vi "Choose Implementation Dialog.vi"(8 "error in (no error)":errorcluster, 9 "DNL_Activate BD":bool, 10 "Method Name":string, 11 "DNL_Wired Class Refnum":refnum<vi>) -> (0 "error out":errorcluster, 2 "Class Hierarchy":string[](array[string]), 3 "DNL_Wired Class Refnum out":refnum<vi>)   [LabVIEW 2020, in "Choose Implementation Dialog.lvlib"]
uses:
  Choose Implementation Dialog.lvlib
  da94b13a-eb72-4d8b-8881-ae04a75001f9.vi
panel:
  in  "format string":string="Error %d while initializing Choose Implementation dialog."
  in  "Class Hierarchy":string[](tree) caption="Select VI"
  in  "Help":bool
  in  "Cancel":bool
  in  "Open":bool
  # "* You can Ctrl-click multiple items in the list to open multiple method VIs."
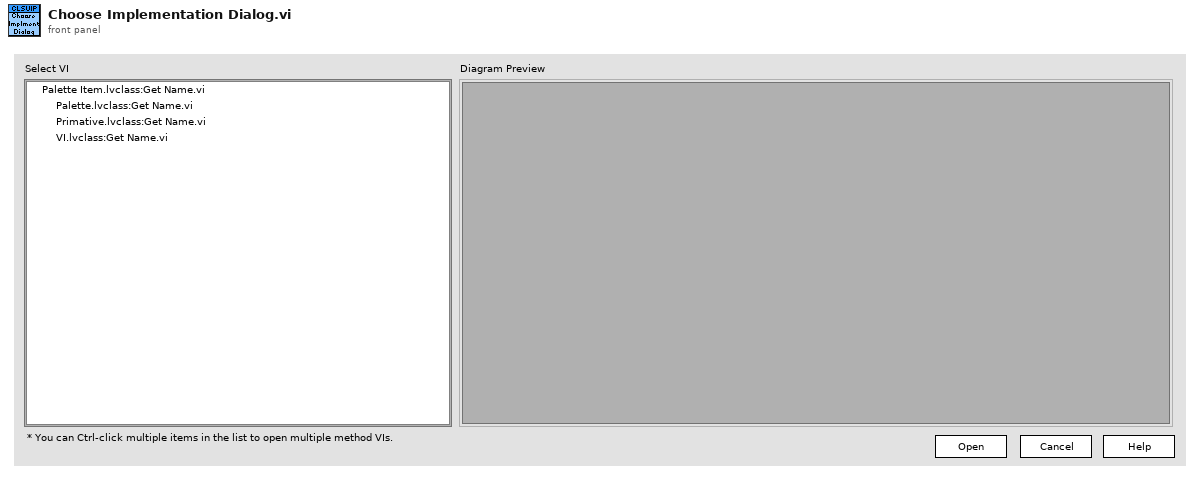
[diagram p1: front panel]
types:
  T1 = typedef "LVPointTypeDef.ctl" = cluster{"Horizontal":i16, "Vertical":i16}
  T2 = typedef "LVRectTypeDef.ctl" = cluster{"Left":i16, "Top":i16, "Right":i16, "Bottom":i16}
  T3 = typedef "LVPoint32TypeDef.ctl" = cluster{"Horizontal":i32, "Vertical":i32}
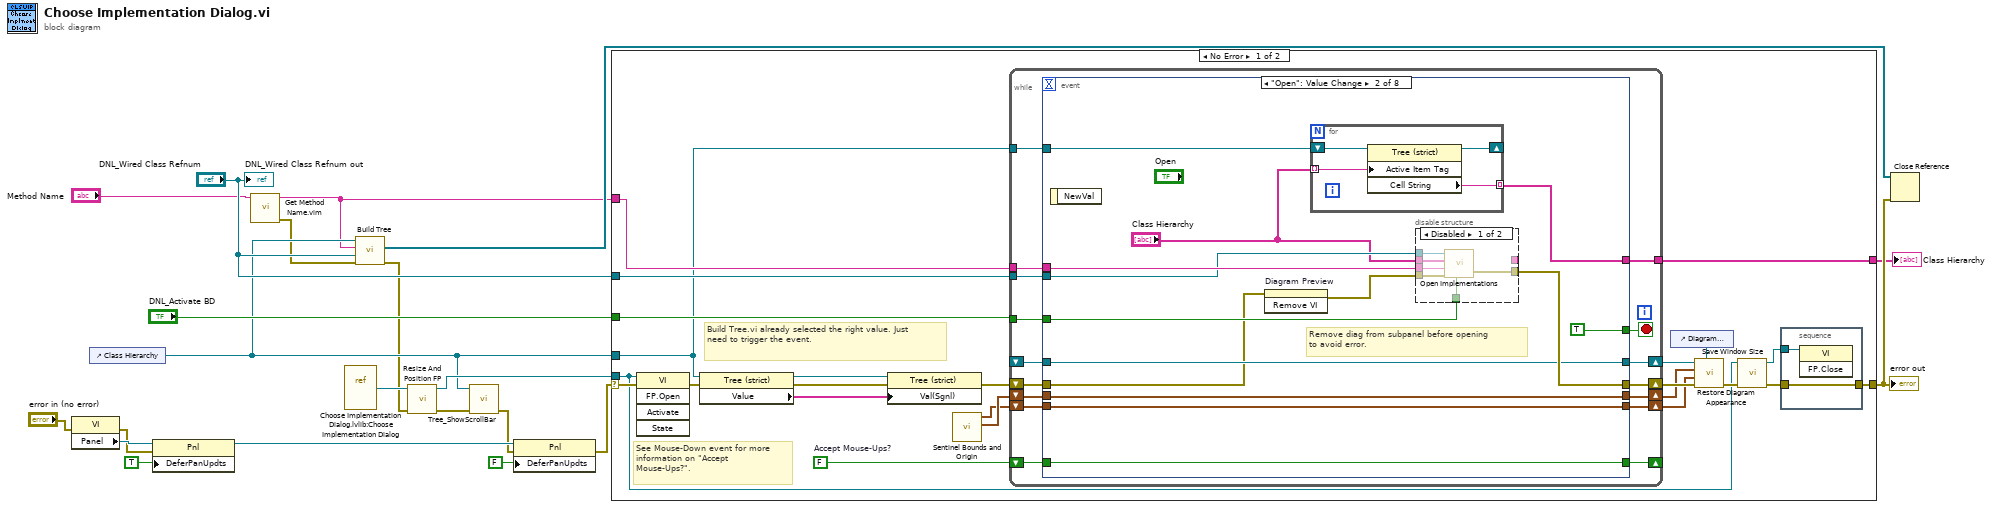
[diagram p0: block diagram]
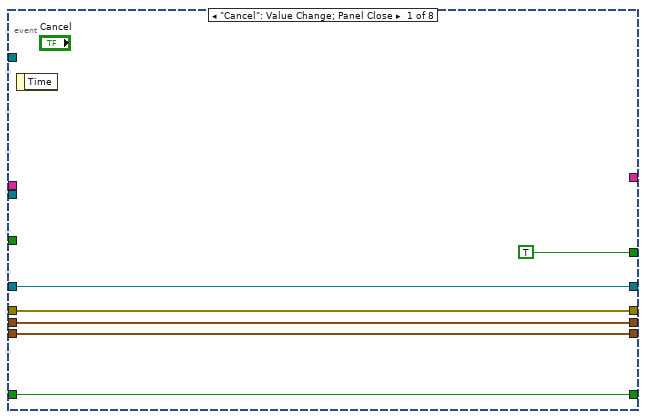
[diagram p2: hidden frame]
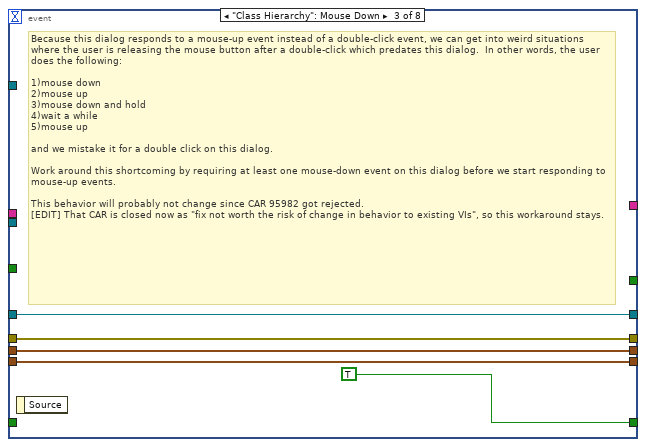
[diagram p4: hidden frame]
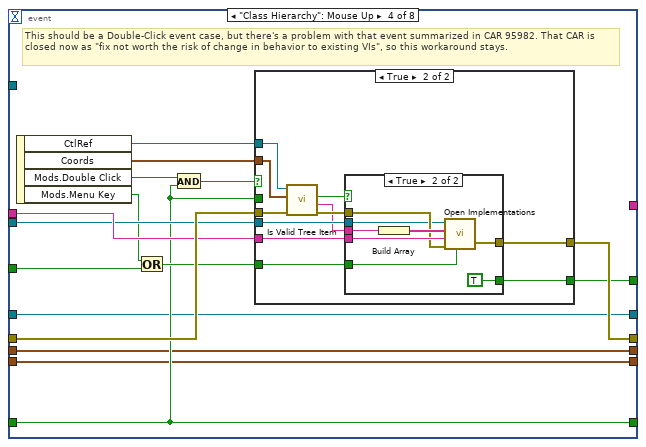
[diagram p5: hidden frame]
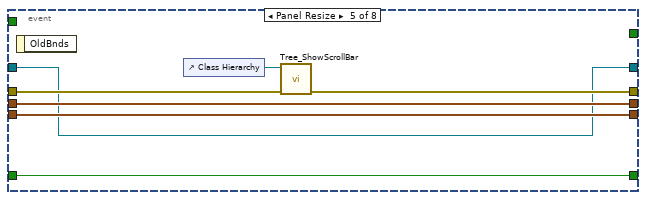
[diagram p8: hidden frame]
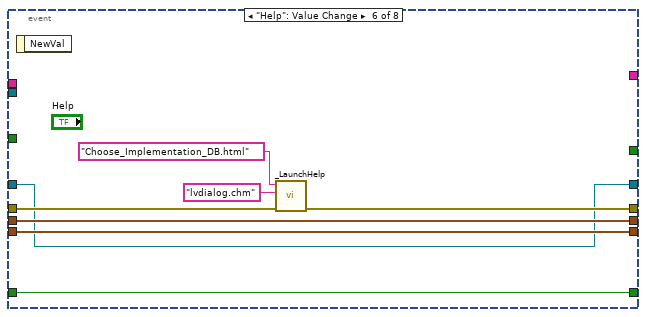
[diagram p9: hidden frame]
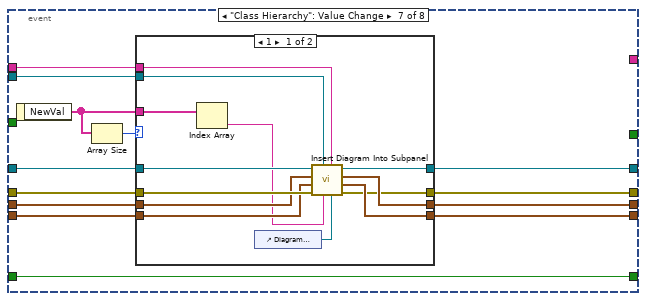
[diagram p10: hidden frame]
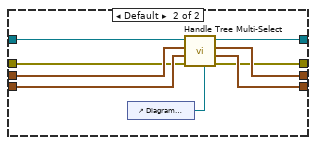
[diagram p11: hidden frame]
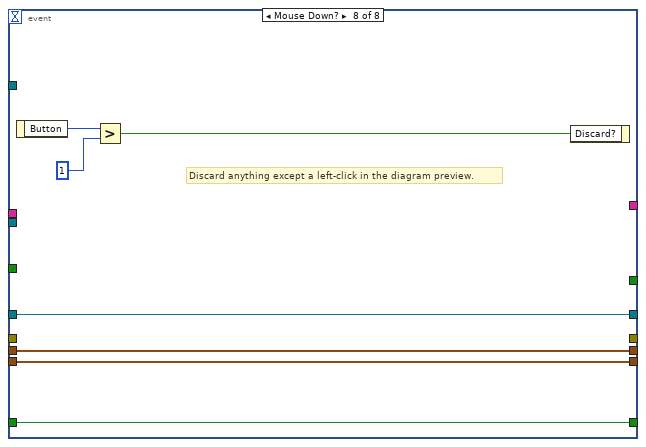
[diagram p12: hidden frame]
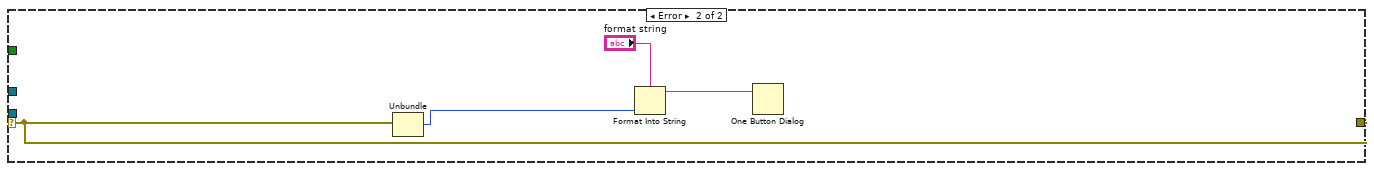
[diagram p13: hidden frame]
diagram:
  n1 = property class="VI"(error in="error in (no error)") -> (error out=w13:errorcluster, "Panel"=w16:refnum<vi>)  [unwired: 1 in, 1 out]
  n2 = control-ref of="Class Hierarchy"() -> (w7:refnum<vi>)
  n3 = property class="Pnl"(reference=w16, error in=w13, "DeferPanUpdts"=TRUE ("Defer Panel Updates")) -> (reference out=w11:refnum<vi>)  [unwired: 1 out]
  n4 = call "Get Method Name.vim"("VI Reference/Name"="Method Name") -> ("error out"=w3:errorcluster, "Method Name"=w2:string)  [unwired: 9 in]
  n5 = vi-ref "Choose Implementation Dialog.lvlib:Choose Implementation Dialog.vi"() -> (w21:refnum<vi>)
  n6 = call "Build Tree.vi"("error in (no error)"=w3, "Wired-in Class Refnum"="DNL_Wired Class Refnum", "Method Name"=w2, "Tree Refnum"=w7) -> ("error out"=w6:errorcluster, "All Classes"=w18:refnum<vi>[])  [unwired: 6 out]
  n7 = call "Resize And Position FP.vi"("error in (no error)"=w6, "VI Reference"=w21) -> ("error out"=w8:errorcluster, "VI Reference out"=w20:refnum<vi>)  [unwired: 8 out]
  n8 = call <vilib>:"Tree_ShowScrollBar.vi"("error in (no error)"=w8, "Tree"=w7) -> ("error out"=w5:errorcluster)  [unwired: 9 in]
  n9 = property class="Pnl"(reference=w11, error in=w5, "DeferPanUpdts"=FALSE ("Defer Panel Updates")) -> (error out=w10:errorcluster)  [unwired: 1 out]
  n10 = case shown="No Error" w10 {
    selector: w10 -> [w44 w195]
    tunnel: w2 -> [w31 _]
    tunnel: w20 -> [w33 _]
    tunnel: [w42 w195] -> w17
    tunnel: "DNL_Wired Class Refnum" -> [w30 _]
    tunnel: "DNL_Activate BD" -> [w39 _]
    tunnel: w7 -> [w22 _]
    tunnel: [w23 _] -> w1
    frame No Error {
      w43 = FALSE  # Accept Mouse-Ups?
      # "Build Tree.vi already selected the right value. Just need to trigger the event."
      # "See Mouse-Down event for more information on \"Accept Mouse-Ups?\"."
      n11 = invoke class="VI" method="FP.Open"(reference=w33, error in=w44) -> (error out=w29:errorcluster)  [unwired: 3 in, 4 out]
      n12 = property class="Tree (strict)"(reference=w22, error in=w29) -> (reference out=w27:refnum<vi>, error out=w28:errorcluster, "Value"=w24:string[])
      n13 = property class="Tree (strict)"(reference=w27, error in=w28, "Val(Sgnl)"=w24) -> (error out=w40:errorcluster)  [unwired: 1 out]
      n14 = call "Sentinel Bounds and Origin.vi"() -> ("Sentinel Origin"=w26:T1, "Sentinel Bounds"=w25:T2)  [unwired: 10 in]
      n15 = while {
        shift-right: [w48] -> w38
        shift-left: w40 -> [w60]
        tunnel: w31 -> [w59]
        tunnel: w39 -> [w58]
        tunnel: w30 -> [w57]
        shift-right: [w55] -> _
        shift-left: w43 -> [w56]
        shift-right: [w51] -> w35
        shift-left: w25 -> [w54]
        shift-right: [w52] -> w36
        shift-left: w26 -> [w53]
        shift-right: [w49] -> w34
        shift-left: _ -> [w50]
        tunnel: [w47] -> w23
        tunnel: w22 -> [w46]
        stop <- w61 stop-if-true
        n16 = event shown="[1] \"Open\": Value Change" {
          selector: _ -> [_ _ _ _ _ _ _ _]
          dyn-events: _ -> [_ _ _ _ _ _ _ _]
          timeout: _ -> [_ _ _ _ _ _ _ _]
          tunnel: [TRUE ("Open") TRUE ("Open") _ w108 _ _ _ _] -> w61
          tunnel: w60 -> [w67 w72 w97 w112 w140 w147 w160 _]
          tunnel: w59 -> [_ w81 _ w111 _ _ w153 _]
          tunnel: w58 -> [_ w80 _ w104 _ _ _ _]
          tunnel: w57 -> [_ w78 _ w110 _ _ w154 _]
          tunnel: [w65 w77 TRUE w102 w142 w146 w158 w192] -> w55
          tunnel: w56 -> [w65 w77 _ w102 w142 w146 w158 w192]
          tunnel: w54 -> [w63 w74 w95 w99 w137 w144 w156 w190]
          tunnel: w53 -> [w64 w75 w96 w100 w138 w145 w157 w191]
          tunnel: [w64 w75 w96 w100 w138 w145 w162 w191] -> w52
          tunnel: [w63 w74 w95 w99 w137 w144 w163 w190] -> w51
          tunnel: w50 -> [w62 w73 w94 w101 w136 w143 w155 w189]
          tunnel: [w62 w73 w94 w101 w136 w143 w161 w189] -> w49
          tunnel: [w67 w76 w97 w109 w141 w148 w159 _] -> w48
          tunnel: [_ w68 _ _ _ _ _ _] -> w47
          tunnel: w46 -> [_ w70 _ _ _ _ _ _]
          event "Cancel": Value Change; Panel Close {
            n17 = event-data() -> ()  [unwired: 2 out]
          }
          event "Open": Value Change {
            # "Remove diag from subpanel before opening\nto avoid error."
            n18 = event-data() -> ()  [unwired: 2 out]
            n19 = invoke on="Diagram Preview" class="SubPnl" method="Remove VI"(error in=w72) -> (error out=w71:errorcluster)  [unwired: 2 in, 2 out]
            n20 = for {
              shift-right: [w82] -> _
              shift-left: w70 -> [w85]
              tunnel: "Class Hierarchy" -> [w84] mode=indexing
              tunnel: [w83] -> w68 mode=indexing
              n21 = property class="Tree (strict)"(reference=w85, "Active Item Tag"=w84) -> (reference out=w82:refnum<vi>, "Cell String"=w83:string)  [unwired: 1 in, 1 out]
            }
            n22 = disable-structure shown="Disabled" {
              disable-tunnel: "Class Hierarchy" -> [w91 w93]
              disable-tunnel: w81 -> [w90 _]
              disable-tunnel: w80 -> [w89 _]
              disable-tunnel: w78 -> [w88 _]
              disable-tunnel: [w87 w92] -> w76
              disable-tunnel: w71 -> [w86 w92]
              disable-tunnel: [_ w93] -> _
              frame Disabled {
                n23 = call "Open Implementations.vi"("Class in"=w88, "Implementation List"=w91, "Method Name"=w90, "error in (no error)"=w86, "Activate BD"=w89) -> ("error out"=w87:errorcluster)  [unwired: 1 out]
              }
              frame Enabled {
              }
            }
          }
          event "Class Hierarchy": Mouse Down {
            # "Because this dialog responds to a mouse-up event instead of a double-click event, we can get into weird situations where the user is releasing the mouse button after a double-click which predates this dialog.  In other words, the user does the following:\n\n1)mouse down\n2)mouse up\n3)mouse down and hold\n4)wait a while\n5)mouse up\n\nand we mistake it for a double click on this dialog.  \n\nWork around this shortcoming by requiring at least one mouse-down event on this dialog before we start responding to mouse-up events.\n\nThis behavior will probably not change since CAR 95982 got rejected. \n[EDIT] That CAR is closed now as \"fix not worth the risk of change in behavior to existing VIs\", so this workaround stays."
            n24 = event-data() -> ()  [unwired: 2 out]
          }
          event "Class Hierarchy": Mouse Up {
            # "This should be a Double-Click event case, but there's a problem with that event summarized in CAR 95982. That CAR is closed now as \"fix not worth the risk of change in behavior to existing VIs\", so this workaround stays."
            n25 = event-data() -> ("CtlRef"=w114:refnum<vi>, "Coords"=w113:T3, "Mods.Double Click"=w107:bool, "Mods.Menu Key"=w105:bool)  [unwired: 1 out]
            n26 = Or(x=w105, y=w104) -> (x .or. y?=w103:bool)
            n27 = And(x=w107, y=w102) -> (x .and. y?=w106:bool)
            n28 = case shown="True" w106 {
              tunnel: w114 -> [_ w126]
              tunnel: w113 -> [_ w125]
              tunnel: w112 -> [w115 w124]
              tunnel: w111 -> [_ w123]
              tunnel: w110 -> [_ w121]
              tunnel: w103 -> [_ w120]
              tunnel: [w115 w119] -> w109
              tunnel: [_ w118] -> w108
              tunnel: w102 -> [_ _]
              frame False {
              }
              frame True {
                n29 = call "Is Valid Tree Item.vi"("error in (no error)"=w124, "Coords"=w125, "TreeRef"=w126) -> ("error out"=w122:errorcluster, "Tag"=w116:string, "Valid Item Selected?"=w117:bool)  [unwired: 6 out]
                n30 = case shown="True" w117 {
                  tunnel: w123 -> [_ w134]
                  tunnel: w122 -> [w127 w133]
                  tunnel: w121 -> [_ w132]
                  tunnel: w120 -> [_ w131]
                  tunnel: [w127 w130] -> w119
                  tunnel: [_ TRUE] -> w118
                  tunnel: w116 -> [_ w128]
                  frame False {
                  }
                  frame True {
                    n31 = Build Array(w128) -> (w135:string[])
                    n32 = call "Open Implementations.vi"("Class in"=w132, "Implementation List"=w135, "Method Name"=w134, "error in (no error)"=w133, "Activate BD"=w131) -> ("error out"=w130:errorcluster)  [unwired: 1 out]
                  }
                }
              }
            }
          }
          event Panel Resize {
            n33 = event-data() -> ()  [unwired: 2 out]
            n34 = control-ref of="Class Hierarchy"() -> (w139:refnum<vi>)
            n35 = call <vilib>:"Tree_ShowScrollBar.vi"("error in (no error)"=w140, "Tree"=w139) -> ("error out"=w141:errorcluster)  [unwired: 9 in]
          }
          event "Help": Value Change {
            n36 = event-data() -> ()  [unwired: 2 out]
            n37 = call <helpdir>:"_LaunchHelp.vi"("error in (no error)"=w147, "CHM or HLP filename (lvdialog.chm)"="lvdialog.chm" ("Help File Name"), "HTML filename"="Choose_Implementation_DB.html" ("String to search for")) -> ("error out"=w148:errorcluster)  [unwired: 4 out]
          }
          event "Class Hierarchy": Value Change {
            n38 = event-data() -> ("NewVal"=w152:string[])  [unwired: 1 out]
            n39 = Array Size(array=w152) -> (size(s)=w151:i32)
            n40 = case shown="1" w151 {
              tunnel: [w176 w182] -> w163
              tunnel: [w175 w184] -> w162
              tunnel: [w174 w178] -> w161
              tunnel: w160 -> [w173 w181]
              tunnel: [w172 w180] -> w159
              tunnel: w157 -> [w171 w185]
              tunnel: w156 -> [w170 w183]
              tunnel: w155 -> [w169 w179]
              tunnel: w154 -> [w166 _]
              tunnel: w153 -> [w165 _]
              tunnel: w152 -> [w164 _]
              frame 1 {
                n41 = Index Array(array=w164) -> (element=w167:string)  [unwired: 1 in]
                n42 = control-ref of="Diagram Preview"() -> (w168:refnum<vi>)
                n43 = call "Insert Diagram Into Subpanel.vi"("Subpanel"=w168, "Method Name"=w165, "Tag"=w167, "Class"=w166, "error in (no error)"=w173, "Bounds in"=w170, "Origin in"=w171, "Old VI"=w169) -> ("error out"=w172:errorcluster, "Bounds out"=w176:T2, "Origin out"=w175:T1, "New VI"=w174:refnum<vi>)
              }
              frame Default {
                n44 = control-ref of="Diagram Preview"() -> (w177:refnum<vi>)
                n45 = call "Handle Tree Multi-Select.vi"("Subpanel"=w177, "error in (no error)"=w181, "Bounds in"=w183, "Origin in"=w185, "Old VI"=w179) -> ("error out"=w180:errorcluster, "Bounds out"=w182:T2, "Origin out"=w184:T1, "New VI"=w178:refnum<vi>)  [unwired: 3 in]
              }
            }
          }
          event Mouse Down? {
            # "Discard anything except a left-click in the diagram preview."
            n46 = event-data() -> ("Button"=w188:u16)  [unwired: 1 out]
            n47 = Greater?(x=w188, y=u16 1) -> (0:w186:bool)
            n48 = event-data("Discard?"=w186) -> ()  [unwired: 1 in, 1 out]
          }
        }
      }
      n49 = control-ref of="Diagram Preview"() -> (w32:refnum<vi>)
      n50 = call "Restore Diagram Appearance.vi"("Subpanel"=w32, "error in (no error)"=w38, "Bounds"=w35, "Origin"=w36, "Inserted VI"=w34) -> ("error out"=w37:errorcluster)  [unwired: 6 in]
      n51 = call "Save Window Size.vi"("error in (no error)"=w37, "VI Reference"=w33) -> ("error out"=w41:errorcluster, "VI Reference out"=w45:refnum<vi>)  [unwired: 8 out]
      n52 = stacked-sequence {
        tunnel: w45 -> [w194]
        tunnel: [w193] -> w42
        tunnel: w41 -> [w193]
        frame #0 {
          n53 = invoke class="VI" method="FP.Close"(reference=w194) -> ()  [unwired: 2 in, 3 out]
        }
      }
    }
    frame Error {
      n54 = Unbundle(w195) -> ("code"=w198:i32)  [unwired: 2 out]
      n55 = Format Into String(format string="format string", w198) -> (resulting string=w196:string)  [unwired: 2 in, 1 out]
      n56 = One Button Dialog(message=w196) -> ()  [unwired: 2 out]
    }
  }
  "error out" <- w17
  "Class Hierarchy" <- w1
  n57 = Close Reference(reference=w18, error in (no error)=w17) -> ()  [unwired: 1 out]
  "DNL_Wired Class Refnum out" <- "DNL_Wired Class Refnum"
